vi "uti_Get cluster elmts refs.vi"(8 "entrée d'erreur (pas d'erreur)":errorcluster, 11 "Cluster ref in":refnum<vi>) -> (0 "error out":errorcluster, 2 "Controls[]":refnum<vi>[](array[refnum]), 3 "Cluster ref out":refnum<vi>)   [LabVIEW 2020, in "UI_Actor.lvlib" / "UI_Actor.lvclass"]
uses:
  UI_Actor.lvclass
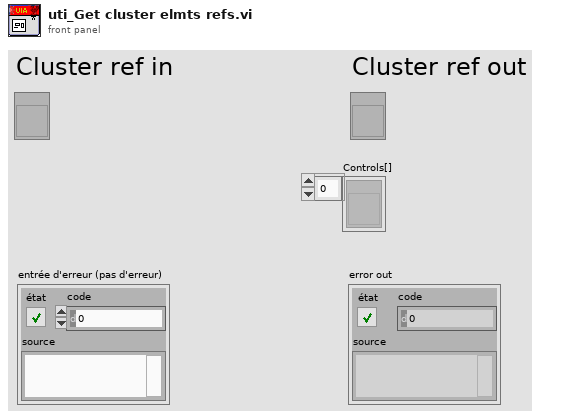
[diagram p1: front panel]
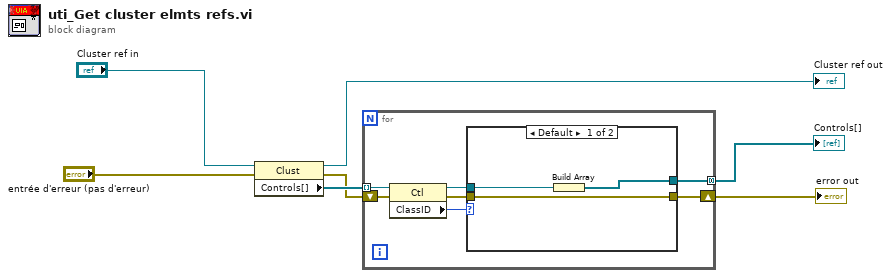
[diagram p0: block diagram]
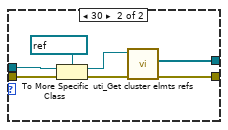
[diagram p2: hidden frame]
diagram:
  n1 = property class="Clust"(reference="Cluster ref in", error in="entrée d'erreur (pas d'erreur)") -> (reference out=→"Cluster ref out":refnum<vi>, error out=w6:errorcluster, "Controls[]"=w7:refnum<vi>[])
  n2 = for {
    tunnel: w7 -> [w14] mode=indexing
    shift-right: [w9] -> w2
    shift-left: w6 -> [w13]
    tunnel: [w10] -> w1 mode=concatenating
    n3 = property class="Ctl"(reference=w14, error in=w13) -> (reference out=w11:refnum<vi>, error out=w8:errorcluster, "ClassID"=w12:u32)
    n4 = case shown="Default" w12 {
      tunnel: [w16 w20] -> w10
      tunnel: w11 -> [w17 w23]
      tunnel: [w15 w19] -> w9
      tunnel: w8 -> [w15 w24]
      frame Default {
        n5 = Build Array(w17) -> (w16:refnum<vi>[])
      }
      frame 30 {
        n6 = To More Specific Class(target class=refnum<vi> refnum ("Cluster"), reference=w23, error in=w24) -> (specific class reference=w18:refnum<vi>, error out=w21:errorcluster)
        n7 = call "uti_Get cluster elmts refs.vi"("entrée d'erreur (pas d'erreur)"=w21, "Cluster ref in"=w18) -> ("error out"=w19:errorcluster, "Controls[]"=w20:refnum<vi>[])  [unwired: 7 in, 1 out]
      }
    }
  }
  "error out" <- w2
  "Controls[]" <- w1
